vi "Demo.vi"() -> ()   [LabVIEW 2016]
uses:
  <userlib>/TSPopup/TSPopup.Popup Cluster.ctl
  <userlib>/TSPopup/TSPopup.lvclass
  <userlib>/TSPopup/TSPopup.Popup Call Parameters.ctl
  <userlib>/TSPopup/TSPopup.Data Type.ctl
panel:
  in  "Popups":T1 {"Boolean" items=["False", "True"]; "Ring" items=["1", "2", "3"]}
  in  "stop":bool
  in  "Signal Settings":i32(listbox)
  # "Type Sensitive\nPopup"
  # "Boolean Colors"
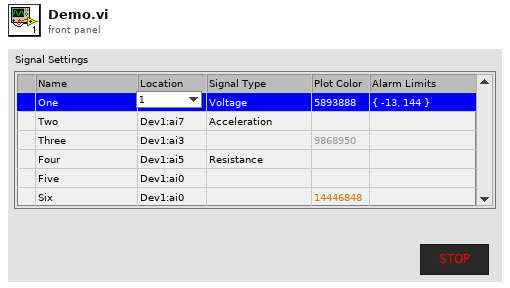
[diagram p1: front panel]
types:
  T1 = typedef "TSPopup.lvlib/TSPopup.lvclass/TSPopup.Popup Cluster.ctl" = cluster{"Unknown":bool, "Unknown 2":bool, "String":string, "Integer":i32, "Float":dbl, "Color":u32, "Boolean":u32, "Ring":u32, "Captioned String":cluster{"String":string, "OK":bool, "Cancel":bool}, "Captioned Integer":cluster{"First":i32, "OK":bool, "Cancel":bool}, "Boolean Colors":cluster{"False":cluster{"FG":u32, "BG":u32}, "True":cluster{"FG":u32, "BG":u32}, "T  to  F":cluster{"FG":u32, "BG":u32}, "F  to  T":cluster{"FG":u32, "BG":u32}, "OK":bool, "Cancel":bool}, "2-Int Cluster":cluster{"First":i32, "Second":i32, "OK":bool, "Cancel":bool}, "4-Int Cluster":cluster{"First":i32, "Second":i32, "Third":i32, "Fourth":i32, "OK":bool, "Cancel":bool}}
  T2 = typedef "TSPopup.lvlib/TSPopup.lvclass/TSPopup.Data Type.ctl" = enum16{"Unkown", "NO POPUP", "String", "Integer", "Float", "Color", "Boolean", "Ring", "Captioned String", "Captioned Integer", "Button Color", "2 Int Cluster", "4 Int Cluster"}
  T3 = typedef "TSPopup.lvlib/TSPopup.lvclass/TSPopup.Popup Call Parameters.ctl" = cluster{"Prop Type":T2, "Initial Value":variant, "Caption Strings":string[], "Ring Strings":string[], "Cell Rect":cluster{"left":i16, "top":i16, "right":i16, "bottom":i16}, "Mouse Coords":cluster{"x":i16, "y":i16}, "Call Data":variant}
  T4 = typedef "LVPoint32TypeDef.ctl" = cluster{"Horizontal":i32, "Vertical":i32}
  T5 = typedef "TSPopup.lvlib/TSPopup.lvclass/TSPopup.Grid.Cell Info.ctl" = cluster{"Tag":string, "Row":i32, "Column":i32, "In Symbol?":bool, "In Data?":bool, "Cell String":string, "Ctl Refnum":refnum<vi>, "Prop Type":T2, "Ring Strings":string[]}
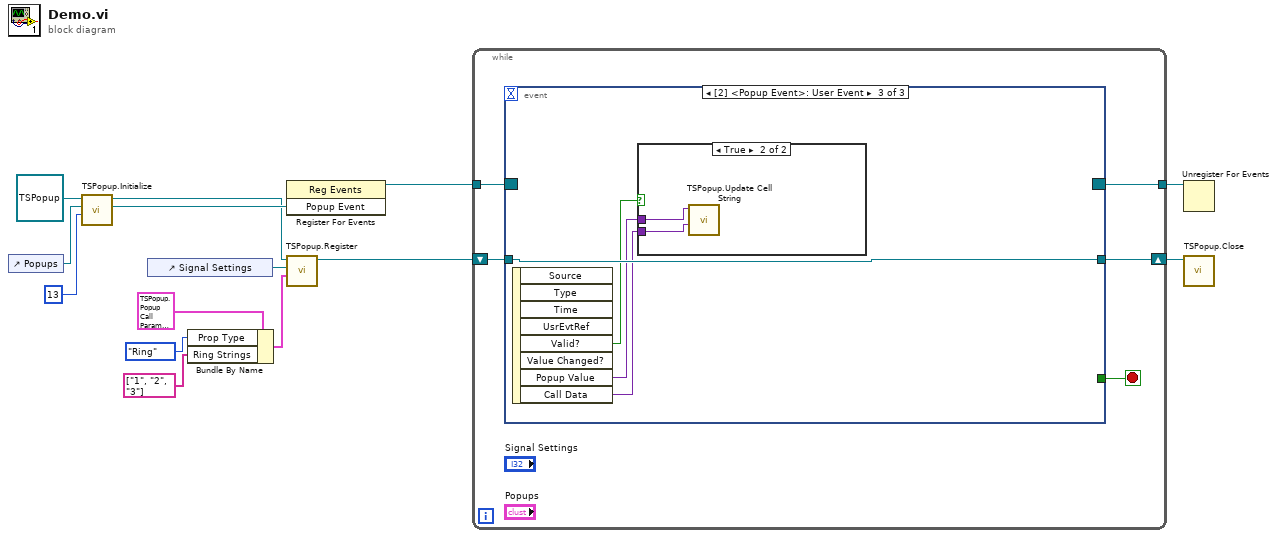
[diagram p0: block diagram]
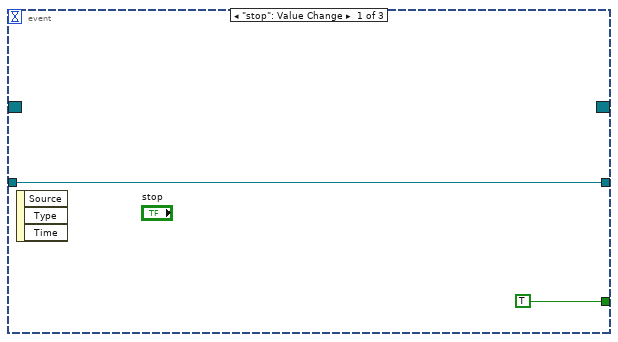
[diagram p2: hidden frame]
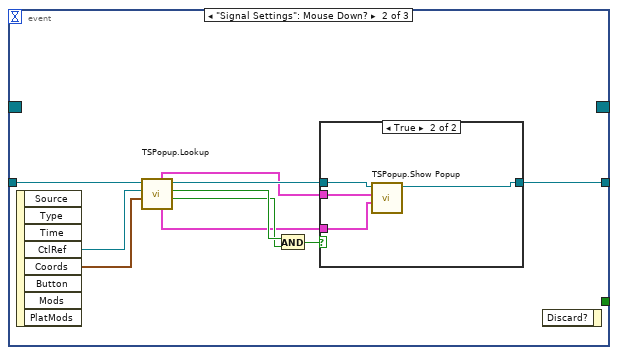
[diagram p3: hidden frame]
diagram:
  n1 = control-ref of="Popups"() -> (w13:refnum<vi>)
  n2 = call <userlib>:"TSPopup.Initialize.vi"("Font Size"=u32 13, "Popup Cluster Ref"=w13, "TSPopup in"=refnum<class "TSPopup.lvclass"> refnum) -> ("Popup Event"=w11:refnum<user-event>, "TSPopup out"=w9:refnum<class "TSPopup.lvclass">)  [unwired: 6 in, 1 out]
  n3 = control-ref of="Signal Settings"() -> (w8:refnum<vi>)
  n4 = Bundle By Name(cluster=T3 {"Prop Type"=enum."String", "Initial Value"=variant, "Caption Strings"=[], "Ring Strings"=[], "Cell Rect"={"left"=0, "top"=0, "right"=0, "bottom"=0}, "Mouse Coords"={"x"=0, "y"=0}, "Call Data"=variant} ("Parameters"), "Prop Type"=TSPopup.Data_Type."Ring", "Ring Strings"=string[] ["1", "2", "3"]) -> (w6:T3)
  n5 = register-events(w11) -> (reference out=w10:refnum<event-registration>)  [unwired: 2 in, 1 out]
  n6 = call <userlib>:"TSPopup.Register.vi"("Parameters"=w6, "Ctl Refnum"=w8, "TSPopup in"=w9) -> ("TSPopup out"=w3:refnum<class "TSPopup.lvclass">)  [unwired: 6 in, 2 out]
  n7 = while {
    tunnel: w10 -> [w19]
    shift-right: [w16] -> w1
    shift-left: w3 -> [w17]
    tunnel: [w15] -> w2
    stop <- w18 stop-if-true
    n8 = event shown="[2] <Popup Event>: User Event" {
      selector: w19 -> [_ _ _]
      dyn-events: [_ _ _] -> w15
      timeout: _ -> [_ _ _]
      tunnel: [TRUE _ _] -> w18
      tunnel: w17 -> [w20 w31 w40]
      tunnel: [w20 w23 w40] -> w16
      event "stop": Value Change {
        n9 = event-data() -> ()  [unwired: 1 in, 3 out]
      }
      event "Signal Settings": Mouse Down? {
        n10 = event-data() -> ("CtlRef"=w30:refnum<vi>, "Coords"=w29:T4)  [unwired: 1 in, 6 out]
        n11 = call <userlib>:"TSPopup.Lookup.vi"("Point"=w29, "Ctl Refnum"=w30, "TSPopup in"=w31) -> ("In Bounds?"=w27:bool, "Found"=w28:bool, "TSPopup out"=w25:refnum<class "TSPopup.lvclass">, "Cell Info (Call data)"=w24:T5, "Popup Parameters"=w22:T3)  [unwired: 3 in, 1 out]
        n12 = And(x=w28, y=w27) -> (x .and. y?=w26:bool)
        n13 = case shown="True" w26 {
          tunnel: w25 -> [w32 w36]
          tunnel: w24 -> [_ w35]
          tunnel: [w32 w34] -> w23
          tunnel: w22 -> [_ w33]
          frame False {
          }
          frame True {
            n14 = call <userlib>:"TSPopup.Show Popup.vi"("Call Data (ignore if empty)"=w35, "Popup Parameters"=w33, "TSPopup in"=w36) -> ("TSPopup out"=w34:refnum<class "TSPopup.lvclass">)  [unwired: 7 in, 1 out]
          }
        }
        n15 = event-data() -> ()  [unwired: 2 in, 1 out]
      }
      event User Event {
        n16 = event-data() -> ("Valid?"=w39:bool, "Popup Value"=w38:variant, "Call Data"=w37:variant)  [unwired: 1 in, 5 out]
        n17 = case shown="True" w39 {
          tunnel: w38 -> [_ w42]
          tunnel: w37 -> [_ w41]
          frame False {
          }
          frame True {
            n18 = call <userlib>:"TSPopup.Update Cell String.vi"("Call Data (must be Cell Info cluster)"=w41, "Popup Value"=w42) -> ()  [unwired: 9 in, 1 out]
          }
        }
      }
    }
  }
  n19 = Unregister For Events(event registration refnum=w2) -> ()  [unwired: 1 in, 1 out]
  n20 = call <userlib>:"TSPopup.Close.vi"("TSPopup in"=w1) -> ()  [unwired: 9 in, 2 out]
